vi "testHexStringByteArrayConversion.vi"(8 "error in (no error)":errorcluster, 11 "TestCase in":refnum<class "TestHexStringConversion.lvclass">) -> (0 "error out":errorcluster, 3 "TestCase out":refnum<class "TestHexStringConversion.lvclass">)   [LabVIEW 2021, in "TestHexStringConversion.lvclass"]
uses:
  TestHexStringConversion.lvclass
  TestHexStringConversion.lvclass/TestHexStringConversion.ctl
  <vilib>/addons/_JKI Toolkits/VI Tester/TestCase.llb/TestCase.lvclass
  Utility/dotNET Crypto Utility.lvlib
  C:/Program Files (x86)/National Instruments/LabVIEW 2021/vi.lib/addons/_JKI Toolkits/VI Tester/TestCase.llb/TestCase.lvclass
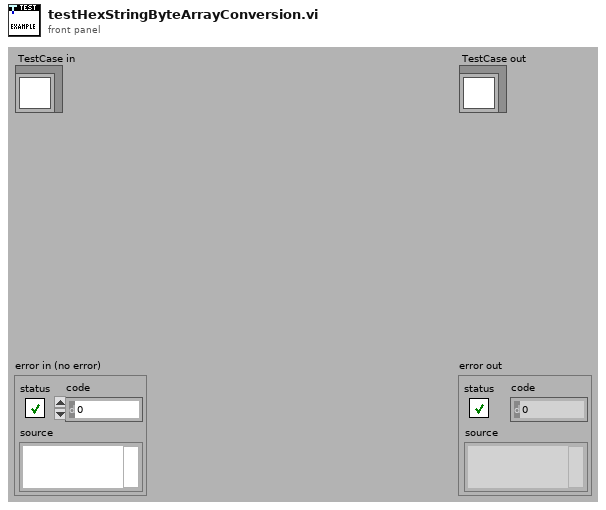
[diagram p1: front panel]
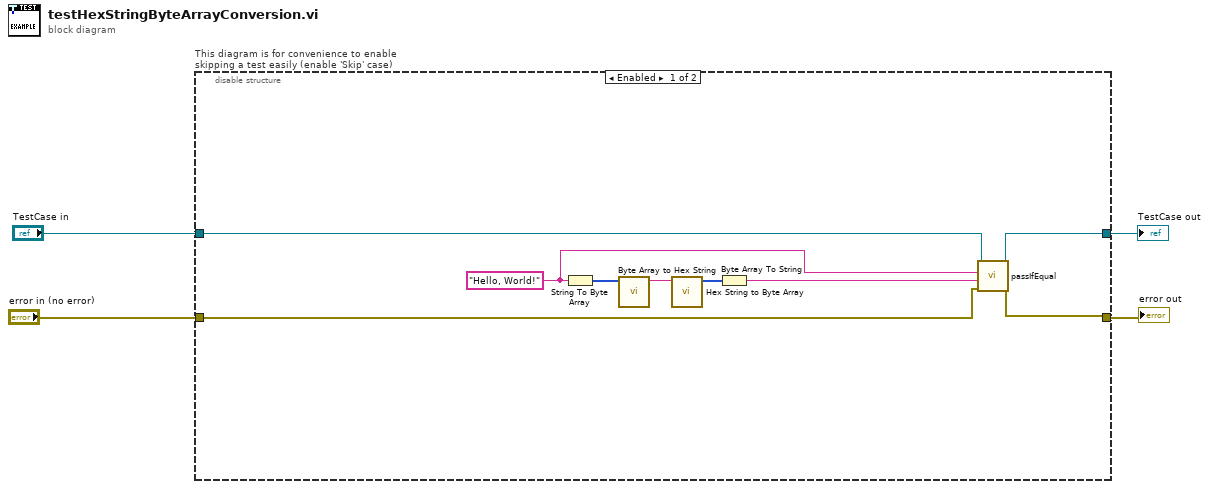
[diagram p0: block diagram]
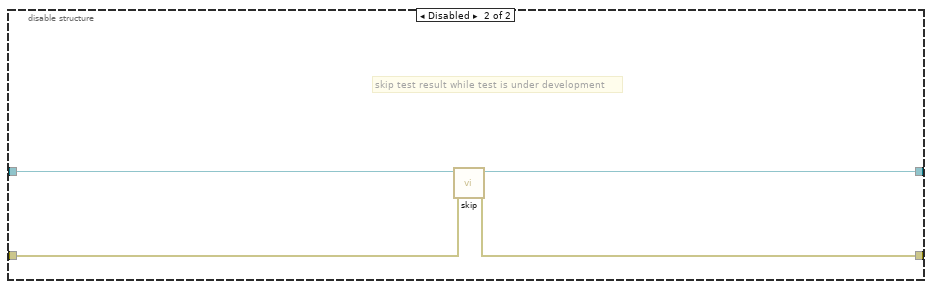
[diagram p2: hidden frame]
diagram:
  n1 = disable-structure "This diagram is for convenience to enable skipping a test easily (enable 'Skip' case)" shown="Enabled" {
    disable-tunnel: "TestCase in" -> [w13 w17]
    disable-tunnel: [w12 w15] -> w1
    disable-tunnel: [w11 w16] -> w3
    disable-tunnel: "error in (no error)" -> [w10 w14]
    frame Enabled {
      w8 = "Hello, World!" ("Hex String")
      n2 = String To Byte Array(string=w8) -> (unsigned byte array=w7:u8[])
      n3 = call "Byte Array to Hex String.vi"("Byte Array"=w7) -> ("Hex String"=w9:string)  [unwired: 10 in]
      n4 = call "Hex String to Byte Array.vi"("Hex String"=w9) -> ("Byte Array"=w6:u8[])  [unwired: 10 in]
      n5 = Byte Array To String(unsigned byte array=w6) -> (string=w5:string)
      n6 = call-dynamic "passIfEqual.vi"("error in (no error)"=w10, "y"=w5, "x"=w8, "TestCase in"=w13) -> ("error out"=w11:errorcluster, "TestCase out"=w12:refnum<class "TestHexStringConversion.lvclass">)  [unwired: 6 in]
    }
    frame Disabled {
      # "skip test result while test is under development"
      n7 = call <vilib>:"skip.vi"("error in (no error)"=w14, "TestCase in"=w17) -> ("error out"=w16:errorcluster, "TestCase out"=w15:refnum<class "TestHexStringConversion.lvclass">)  [unwired: 8 in]
    }
  }
  "error out" <- w3
  "TestCase out" <- w1
